vi "tanh.vi"(0 "x":dbl[][](array[numeric])) -> (7 "y":dbl[][](array[numeric]))   [LabVIEW 2014]
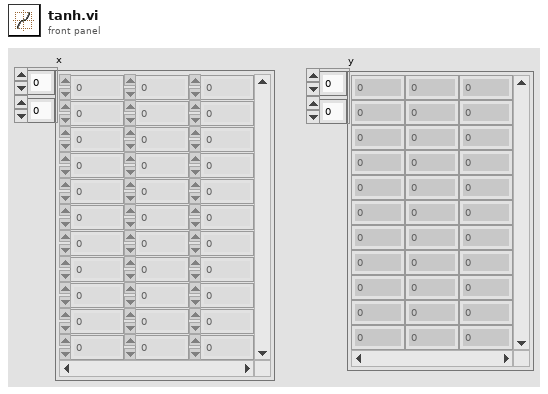
[diagram p1: front panel]
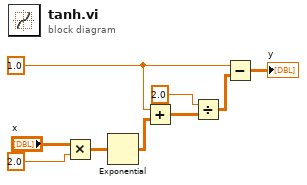
[diagram p0: block diagram]
diagram:
  w3 = 1.0
  n1 = Multiply(x="x", y=2.0) -> (x*y=w7:dbl[][])
  n2 = Exponential(1:w7) -> (0:w6:dbl[][])
  n3 = Add(x=w3, y=w6) -> (x+y=w5:dbl[][])
  n4 = Divide(x=2.0, y=w5) -> (x/y=w2:dbl[][])
  n5 = Subtract(x=w3, y=w2) -> (x-y=→"y":dbl[][])
